vi "SetValueByItemTag.vi"(0 "VI Reference In":refnum<vi>, 2 "delimiter (>>)":string=">>", 5 "Control Path":string, 7 "Item Tag":string, 11 "Error In":errorcluster) -> (4 "VI Reference Out":refnum<vi>, 15 "Error Out":errorcluster)   [LabVIEW 2016, in "Drona.lvlib" / "ControlValue.lvlib" / "StimulusTree.lvlib"]
doc: "Sets value(signaling) for the tree control whose item tag is specified. \n\nThe input control name is given as a string , incase of path, use delimiters inbetween the path."
uses:
  StimulusTree.lvlib
  <vilib>/Utility/error.llb/Error Cluster From Error Code.vi
  <vilib>/ErrorRing/Error Ring.xnode
  Drona.lvlib
  Get/GetControlRef/GetControlRef.lvlib
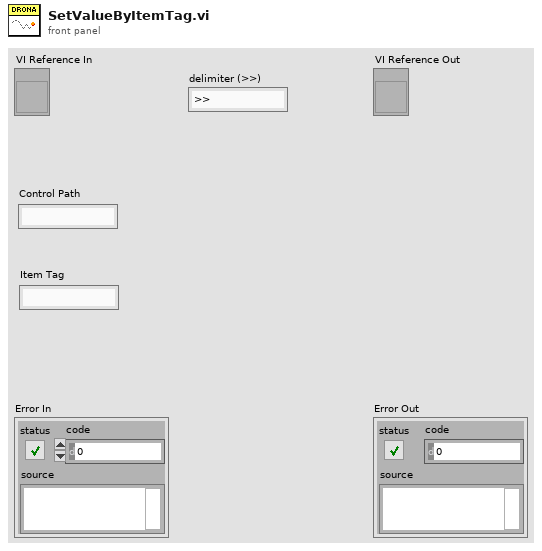
[diagram p1: front panel]
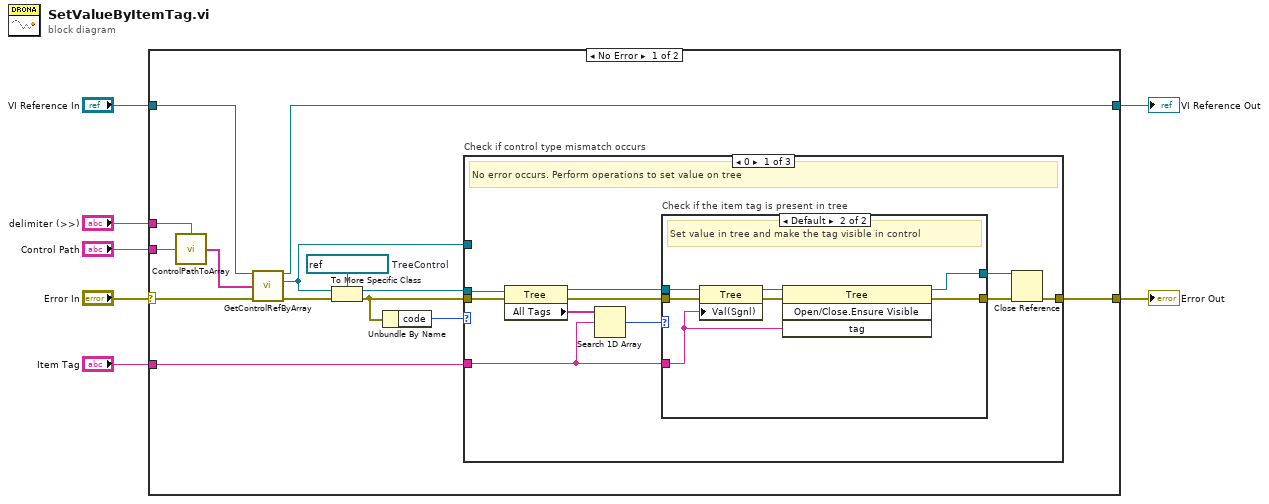
[diagram p0: block diagram]
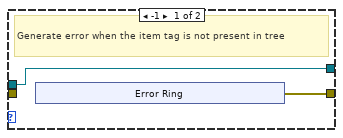
[diagram p2: hidden frame]
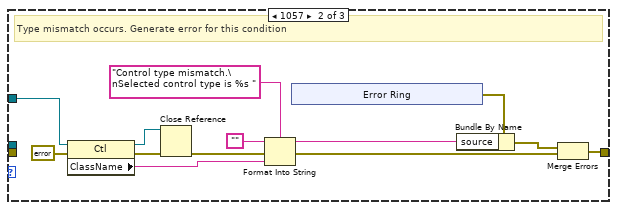
[diagram p3: hidden frame]
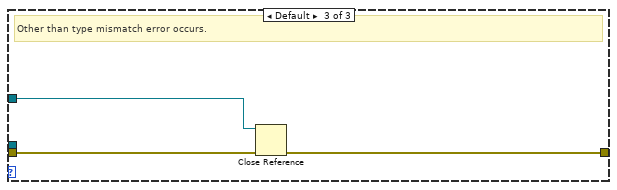
[diagram p4: hidden frame]
diagram:
  n1 = case shown="No Error" "Error In" {
    selector: "Error In" -> [w18 w68]
    tunnel: [w9 w68] -> w6
    tunnel: "VI Reference In" -> [w17 w67]
    tunnel: "Control Path" -> [w20 _]
    tunnel: [w14 w67] -> w3
    tunnel: "delimiter (>>)" -> [w19 _]
    tunnel: "Item Tag" -> [w10 _]
    frame No Error {
      w21 = refnum<vi> refnum  # TreeControl
      n2 = call "ControlPathToArray.vi"("Control Name"=w20, "delimiter (>>)"=w19) -> ("Control Path"=w16:string[])
      n3 = call "GetControlRefByArray.vi"("VI Reference In"=w17, "Control Path"=w16, "error In"=w18) -> ("VI Reference Out"=w14:refnum<vi>, "Ctl Refnum"=w11:refnum<vi>, "error out"=w15:errorcluster)  [unwired: 10 in]
      n4 = To More Specific Class(target class=w21, reference=w11, error in=w15) -> (specific class reference=w12:refnum<vi>, error out=w13:errorcluster)
      n5 = Unbundle By Name(w13) -> ("code"=w8:i32)
      n6 = case "Check if control type mismatch occurs" shown="0" w8 {
        tunnel: [w31 w48 w65] -> w9
        tunnel: w12 -> [w26 _ _]
        tunnel: w10 -> [w22 _ _]
        tunnel: w11 -> [_ w58 w64]
        tunnel: w13 -> [w30 _ w66]
        frame 0 {
          # "No error occurs. Perform operations to set value on tree"
          n7 = property class="Tree"(reference=w26, error in=w30) -> (reference out=w25:refnum<vi>, error out=w27:errorcluster, "All Tags"=w24:string[])
          n8 = Search 1D Array(1D array=w24, element=w22) -> (index of element=w23:i32)  [unwired: 1 in]
          n9 = case "Check if the item tag is present in tree" shown="Default" w23 {
            tunnel: [w32 w42] -> w29
            tunnel: [w33 w39] -> w28
            tunnel: w27 -> [_ w45]
            tunnel: w25 -> [w33 w44]
            tunnel: w22 -> [_ w40]
            frame -1 {
              # "Generate error when the item tag is not present in tree"
              n10 = xnode "Error Ring"() -> ("error out"=w32:errorcluster)
            }
            frame Default {
              # "Set value in tree and make the tag visible in control"
              n11 = property class="Tree"(reference=w44, error in=w45, "Val(Sgnl)"=w40) -> (reference out=w41:refnum<vi>, error out=w43:errorcluster)
              n12 = invoke class="Tree" method="Open/Close.Ensure Visible"(reference=w41, error in=w43, "tag"=w40) -> (reference out=w39:refnum<vi>, error out=w42:errorcluster)  [unwired: 1 in, 2 out]
            }
          }
          n13 = Close Reference(reference=w28, error in (no error)=w29) -> (error out=w31:errorcluster)
        }
        frame 1057 {
          # "Type mismatch occurs. Generate error for this condition"
          n14 = property class="Ctl"(reference=w58, error in=errorcluster {"status"=FALSE, "code"=0, "source"=""} ("error out")) -> (reference out=w46:refnum<vi>, error out=w57:errorcluster, "ClassName"=w54:string)
          n15 = Close Reference(reference=w46, error in (no error)=w57) -> (error out=w47:errorcluster)
          n16 = Format Into String(format string="Control type mismatch.\nSelected control type is %s ", initial string="", error in=w47, w54) -> (resulting string=w51:string, error out=w49:errorcluster)
          n17 = xnode "Error Ring"() -> ("error out"=w52:errorcluster)
          n18 = Bundle By Name(cluster=w52, "source"=w51) -> (w50:errorcluster)
          n19 = Merge Errors(w50, w49) -> (w48:errorcluster)
        }
        frame Default {
          # "Other than type mismatch error occurs."
          n20 = Close Reference(reference=w64, error in (no error)=w66) -> (error out=w65:errorcluster)
        }
      }
    }
    frame Error {
    }
  }
  "Error Out" <- w6
  "VI Reference Out" <- w3
